vi "YAG_init.v5.vi"(8 "error in (no error)":errorcluster, 9 "initial V":dbl=700.0, 10 "initial rep rate":dbl=10.0, 11 "VISA Refnum in":refnum<visa-resource-name>="COM1") -> (0 "error out":errorcluster={"status"=FALSE, "code"=1073676294, "source"="VISA Read in Cmd-Reply.vi->YAG_init.vi->YAG_Control.v2.vi"}, 3 "VISA Refnum out":refnum<visa-resource-name>="COM1")   [LabVIEW 2022 SP3]
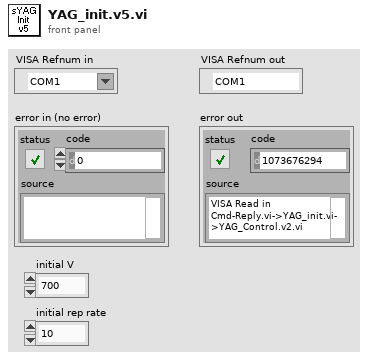
[diagram p1: front panel]
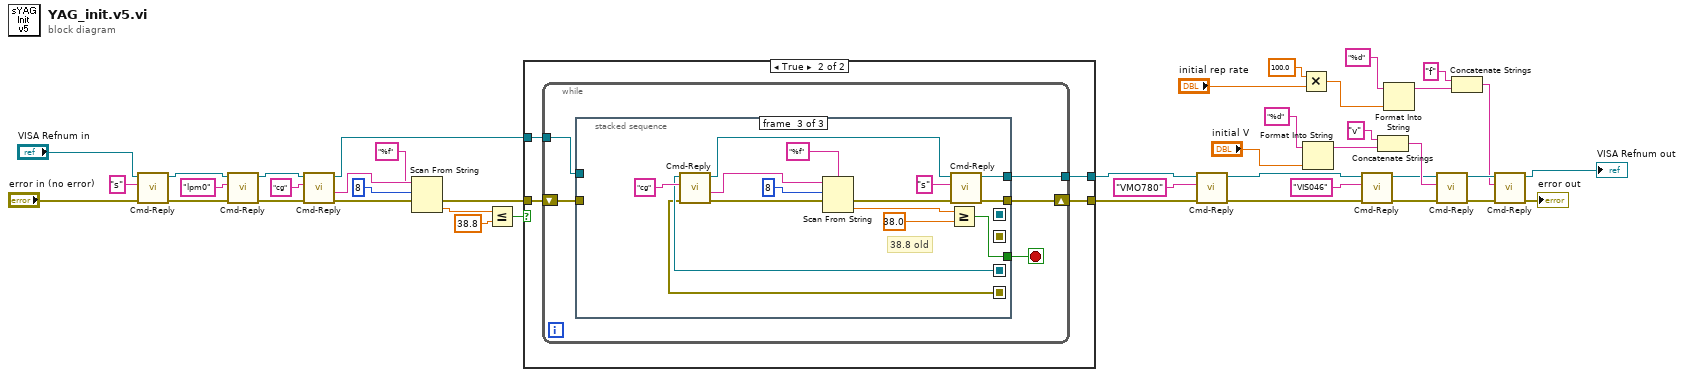
[diagram p0: block diagram]
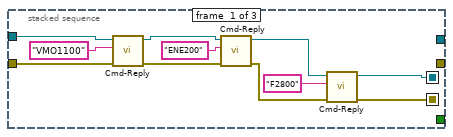
[diagram p3: hidden frame]
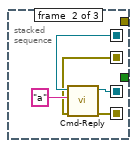
[diagram p4: hidden frame]
diagram:
  n1 = call "Cmd-Reply.vi"("error in (no error)"="error in (no error)", "cmd"="s", "VISA Refnum in"="VISA Refnum in") -> ("error out"=w39:errorcluster, "VISA Refnum out"=w38:refnum<visa-resource-name>)  [unwired: 6 in, 1 out]
  n2 = call "Cmd-Reply.vi"("error in (no error)"=w39, "cmd"="lpm0", "VISA Refnum in"=w38) -> ("error out"=w13:errorcluster, "VISA Refnum out"=w15:refnum<visa-resource-name>)  [unwired: 6 in, 1 out]
  n3 = call "Cmd-Reply.vi"("error in (no error)"=w13, "cmd"="cg" ("write buffer"), "VISA Refnum in"=w15) -> ("error out"=w17:errorcluster, "reply"=w19:string, "VISA Refnum out"=w14:refnum<visa-resource-name>)  [unwired: 6 in]
  n4 = Scan From String(format string="%f", input string=w19, initial scan location=u32 8, error in=w17) -> (error out=w12:errorcluster, output 1=w11:dbl)  [unwired: 1 in, 2 out]
  n5 = Less Or Equal?(x=w11, y=38.8) -> (x <= y?=w9:bool)
  n6 = case shown="True" w9 {
    tunnel: w14 -> [w44 w48]
    tunnel: [w44 w45] -> w4
    tunnel: w12 -> [w43 w47]
    tunnel: [w43 w46] -> w2
    frame False {
    }
    frame True {
      n7 = while {
        tunnel: w48 -> [w53]
        shift-right: [w49] -> w46
        shift-left: w47 -> [w51]
        tunnel: [w50] -> w45
        stop <- w52 stop-if-true
        n8 = stacked-sequence {
          seq-local: [w62 _ _] -> [_ w69 _]
          seq-local: [_ w68 _] -> [_ _ w77]
          seq-local: [w60 _ _] -> [_ w66 _]
          seq-local: [_ w65 _] -> [_ _ w75]
          tunnel: w53 -> [w58 _ _]
          tunnel: [_ _ w76] -> w52
          tunnel: w51 -> [w55 _ _]
          tunnel: [_ _ w72] -> w50
          tunnel: [_ _ w70] -> w49
          frame #0 {
            n9 = call "Cmd-Reply.vi"("error in (no error)"=w55, "cmd"="VMO1100", "VISA Refnum in"=w58) -> ("error out"=w54:errorcluster, "VISA Refnum out"=w57:refnum<visa-resource-name>)  [unwired: 6 in, 1 out]
            n10 = call "Cmd-Reply.vi"("error in (no error)"=w54, "cmd"="ENE200", "VISA Refnum in"=w57) -> ("error out"=w61:errorcluster, "VISA Refnum out"=w63:refnum<visa-resource-name>)  [unwired: 6 in, 1 out]
            n11 = call "Cmd-Reply.vi"("error in (no error)"=w61, "cmd"="F2800", "VISA Refnum in"=w63) -> ("error out"=w60:errorcluster, "VISA Refnum out"=w62:refnum<visa-resource-name>)  [unwired: 6 in, 1 out]
          }
          frame #1 {
            n12 = call "Cmd-Reply.vi"("error in (no error)"=w66, "cmd"="a", "VISA Refnum in"=w69) -> ("error out"=w65:errorcluster, "VISA Refnum out"=w68:refnum<visa-resource-name>)  [unwired: 6 in, 1 out]
          }
          frame #2 {
            # "38.8 old"
            n13 = call "Cmd-Reply.vi"("error in (no error)"=w75, "cmd"="cg" ("write buffer"), "VISA Refnum in"=w77) -> ("error out"=w81:errorcluster, "reply"=w83:string, "VISA Refnum out"=w73:refnum<visa-resource-name>)  [unwired: 6 in]
            n14 = Scan From String(format string="%f", input string=w83, initial scan location=u32 8, error in=w81) -> (error out=w71:errorcluster, output 1=w79:dbl)  [unwired: 1 in, 2 out]
            n15 = Greater Or Equal?(x=w79, y=38.0) -> (x >= y?=w76:bool)
            n16 = call "Cmd-Reply.vi"("error in (no error)"=w71, "cmd"="s", "VISA Refnum in"=w73) -> ("error out"=w70:errorcluster, "VISA Refnum out"=w72:refnum<visa-resource-name>)  [unwired: 6 in, 1 out]
          }
        }
      }
    }
  }
  n17 = call "Cmd-Reply.vi"("error in (no error)"=w2, "cmd"="VMO780" ("concatenated string"), "VISA Refnum in"=w4) -> ("error out"=w5:errorcluster, "VISA Refnum out"=w8:refnum<visa-resource-name>)  [unwired: 6 in, 1 out]
  n18 = Multiply(x=100.0, y="initial rep rate") -> (x*y=w31:dbl)
  n19 = Format Into String(format string="%d", "initial V") -> (resulting string=w36:string)  [unwired: 2 in, 1 out]
  n20 = call "Cmd-Reply.vi"("error in (no error)"=w5, "cmd"="VIS046" ("concatenated string"), "VISA Refnum in"=w8) -> ("error out"=w1:errorcluster, "VISA Refnum out"=w3:refnum<visa-resource-name>)  [unwired: 6 in, 1 out]
  n21 = Concatenate Strings("v" ("string"), w36) -> (w21:string)
  n22 = Format Into String(format string="%d", w31) -> (resulting string=w29:string)  [unwired: 2 in, 1 out]
  n23 = call "Cmd-Reply.vi"("error in (no error)"=w1, "cmd"=w21, "VISA Refnum in"=w3) -> ("error out"=w25:errorcluster, "VISA Refnum out"=w27:refnum<visa-resource-name>)  [unwired: 6 in, 1 out]
  n24 = Concatenate Strings("f" ("string"), w29) -> (w23:string)
  n25 = call "Cmd-Reply.vi"("error in (no error)"=w25, "cmd"=w23, "VISA Refnum in"=w27) -> ("error out"=→"error out":errorcluster, "VISA Refnum out"=→"VISA Refnum out":refnum<visa-resource-name>)  [unwired: 6 in, 1 out]
